vi "Programmatically Export Modify and Import SystemLink State.vi"() -> ()   [LabVIEW 2017]
uses:
  <vilib>/National Instruments/SystemLink Repository API (Beta)/SystemLink_Repo_API.lvlib
  SystemLink_States_API.lvlib
panel:
  in  "Target LabVIEW version for reuse libraries":string
  in  "state name":string
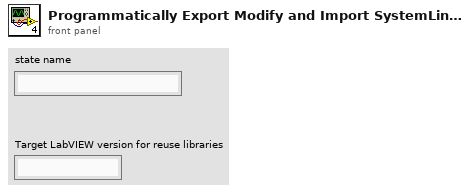
[diagram p1: front panel]
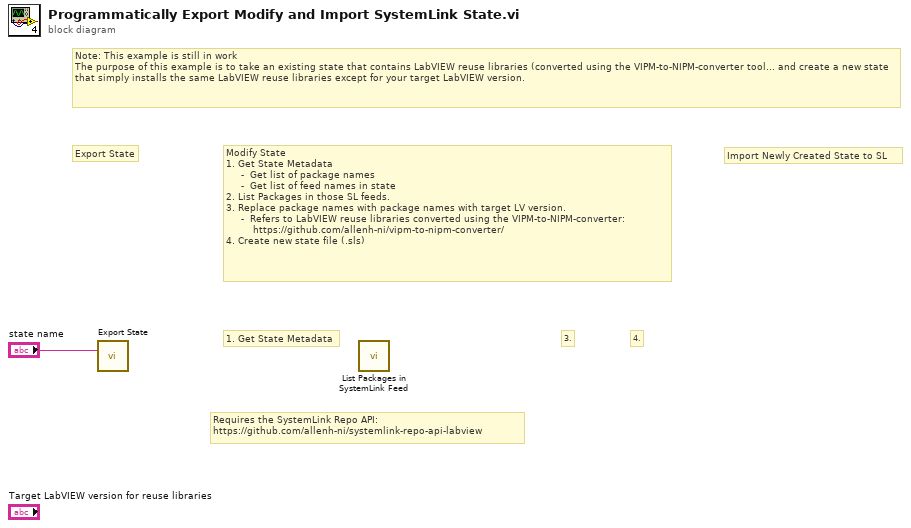
[diagram p0: block diagram]
diagram:
  # "Note: This example is still in work\nThe purpose of this example is to take an existing state that contains LabVIEW reuse libraries (converted using the VIPM-to-NIPM-converter tool... and create a new state that simply installs the same LabVIEW reuse libraries except for your target LabVIEW version."
  # "4."
  # "3."
  # "1. Get State Metadata"
  # "Requires the SystemLink Repo API:\nhttps://github.com/allenh-ni/systemlink-repo-api-labview"
  # "Import Newly Created State to SL"
  # "Modify State\n1. Get State Metadata\n     -  Get list of package names \n     -  Get list of feed names in state\n2. List Packages in those SL feeds.\n3. Replace package names with package names with target LV version.\n     -  Refers to LabVIEW reuse libraries converted using the VIPM-to-NIPM-converter:\n         https://github.com/allenh-ni/vipm-to-nipm-converter/\n4. Create new state file (.sls)"
  # "Export State"
  n1 = call "Export State.vi"("state name"="state name") -> ()  [unwired: 11 in, 4 out]
  n2 = call <vilib>:"List Packages in SystemLink Feed.vi"() -> ()  [unwired: 12 in, 4 out]
